vi "SubVI_ToggleOnRise2_Teleop.vi"(10 "Input":bool) -> (2 "toggled":bool)   [LabVIEW 2017]
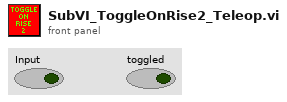
[diagram p1: front panel]
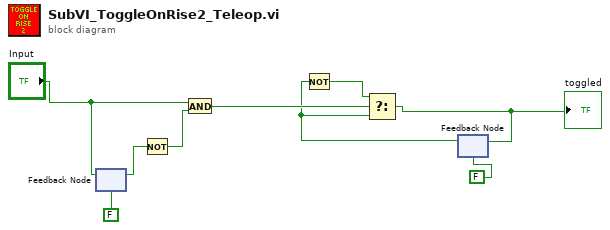
[diagram p0: block diagram]
diagram:
  n1 = feedback #1(FALSE ("Input")) -> (w1:bool)
  n2 = feedback-in #1("Input") -> ()
  n3 = Not(x=w1) -> (.not. x?=w2:bool)
  n4 = And(x="Input", y=w2) -> (x .and. y?=w8:bool)
  n5 = feedback #2(FALSE) -> (w5:bool)
  n6 = Not(x=w5) -> (.not. x?=w4:bool)
  n7 = Select(t=w4, s=w8, f=w5) -> (s? t:f=w3:bool)
  "toggled" <- w3
  n8 = feedback-in #2(w3) -> ()
